vi "Read Info.vi"(8 "error in (no error)":errorcluster, 11 "EventsAbstract in":refnum<class "EventsAbstract.lvclass">) -> (0 "error out":errorcluster, 2 "Info":T1, 3 "EventsAbstract out":refnum<class "EventsAbstract.lvclass">)   [LabVIEW 2019, in "EventsAbstract.lvclass"]
uses:
  EventsAbstract.lvclass
  EventsAbstract.lvclass/EventsAbstract.ctl
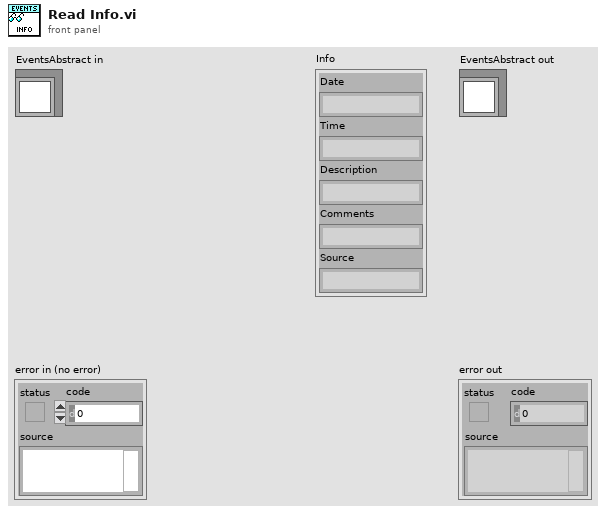
[diagram p1: front panel]
types:
  T1 = cluster{"Date":string, "Time":string, "Description":string, "Comments":string, "Source":string}
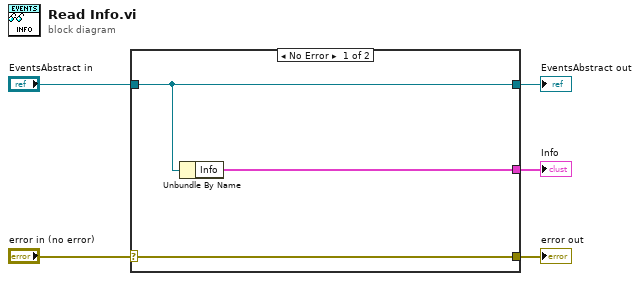
[diagram p0: block diagram]
diagram:
  n1 = case shown="No Error" "error in (no error)" {
    selector: "error in (no error)" -> [w8 w9]
    tunnel: [w8 w9] -> w4
    tunnel: [w7 w10] -> w2
    tunnel: "EventsAbstract in" -> [w7 w10]
    tunnel: [w6 _] -> w1
    frame No Error {
      n2 = Unbundle By Name(w7) -> ("Info"=w6:T1)
    }
    frame Error {
    }
  }
  "error out" <- w4
  "EventsAbstract out" <- w2
  "Info" <- w1
